vi "Get Protection Classes List.vi"(8 "error in (no error)":errorcluster) -> (0 "error out":errorcluster, 2 "Protection names":string[](array[string]), 3 "Class Lookup":variant)   [LabVIEW 2024, in "Instrument Addon Scripting API.lvlib"]
uses:
  Instrument Addon Scripting API.lvlib
  <vilib>/Utility/LVLibp/NI_PackedLibraryUtility.lvlib
  NationalInstruments.VeriStand
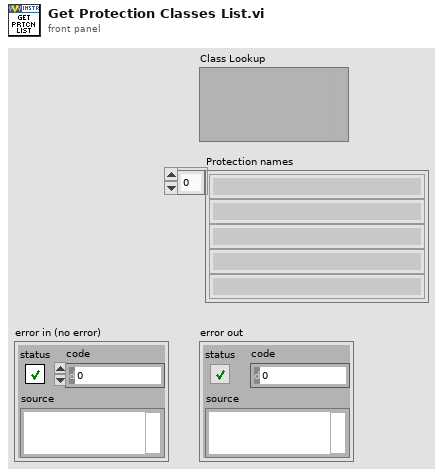
[diagram p1: front panel]
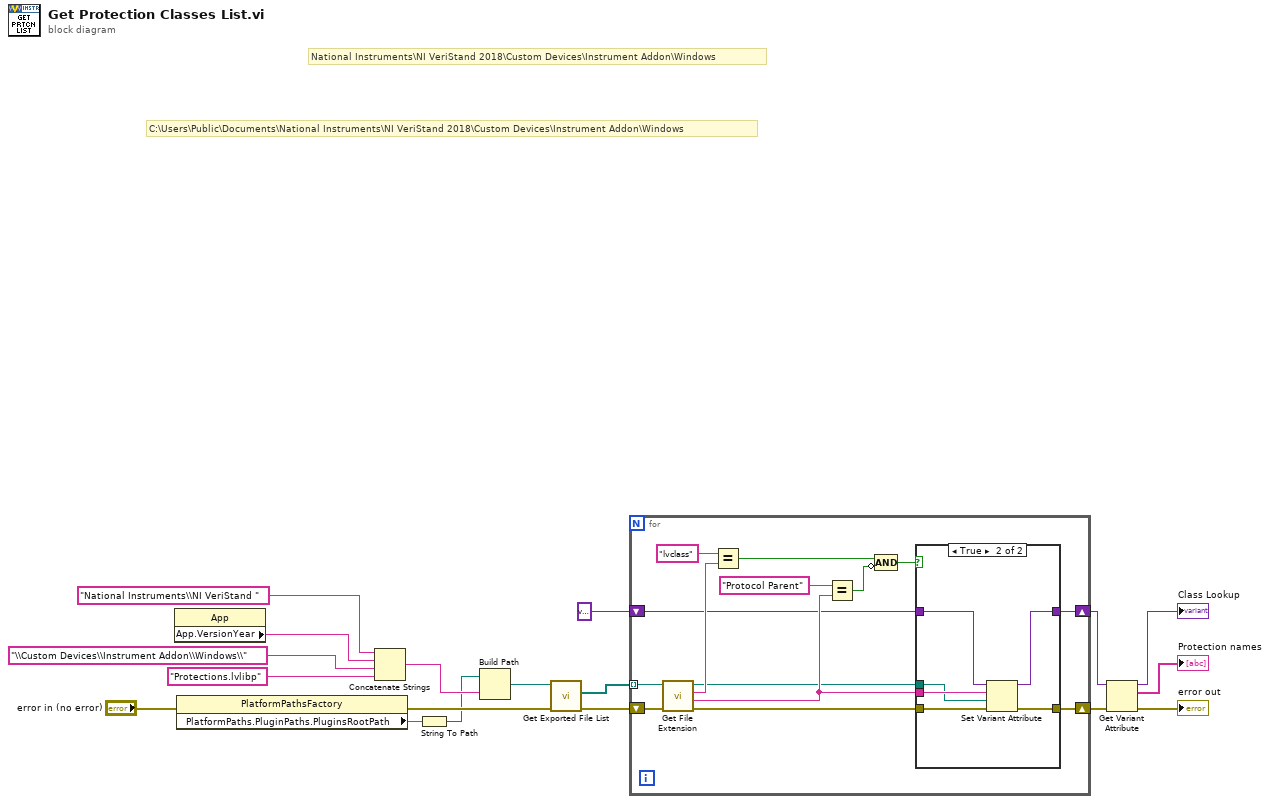
[diagram p0: block diagram]
diagram:
  # "National Instruments\\NI VeriStand 2018\\Custom Devices\\Instrument Addon\\Windows"
  # "C:\\Users\\Public\\Documents\\National Instruments\\NI VeriStand 2018\\Custom Devices\\Instrument Addon\\Windows"
  n1 = property class="App"() -> ("App.VersionYear"=w16:string)  [unwired: 2 in, 2 out]
  n2 = property class="PlatformPathsFactory"(error in="error in (no error)") -> (error out=w4:errorcluster, "PlatformPaths.PluginPaths.PluginsRootPath"=w2:string)  [unwired: 1 in, 1 out]
  n3 = Concatenate Strings("National Instruments\\NI VeriStand " ("string"), w16, "\\Custom Devices\\Instrument Addon\\Windows\\" ("string"), "Protections.lvlibp" ("name or relative path")) -> (w18:string)
  n4 = String To Path(string=w2) -> (path=w1:path)
  n5 = Build Path(base path=w1, name or relative path=w18) -> (appended path=w11:path)
  n6 = call <vilib>:"Get Exported File List.vi"("error in (no error)"=w4, "packed library path"=w11) -> ("error out"=w13:errorcluster, "paths"=w12:path[])  [unwired: 7 in, 1 out]
  n7 = for {
    tunnel: w12 -> [w27] mode=indexing
    shift-right: [w21] -> w8
    shift-left: w13 -> [w28]
    shift-right: [w20] -> w6
    shift-left: variant ("variant") -> [w23]
    n8 = call <vilib>:"Get File Extension.vi"("error in (no error)"=w28, "file"=w27) -> ("error out"=w22:errorcluster, "filename without extension"=w25:string, "lowercase file extension"=w29:string, "dup file"=w24:path)  [unwired: 5 in, 1 out]
    n9 = Equal?(x="lvclass" ("string"), y=w29) -> (x = y?=w31:bool)
    n10 = Equal?(x="Protocol Parent", y=w25) -> (x = y?=w26:bool)
    n11 = Compound Arithmetic op=AND(w31, invert w26) -> (w19:bool)
    n12 = case shown="True" w19 {
      tunnel: w25 -> [_ w40]
      tunnel: w24 -> [_ w39]
      tunnel: w23 -> [w33 w38]
      tunnel: w22 -> [w34 w37]
      tunnel: [w34 w36] -> w21
      tunnel: [w33 w35] -> w20
      frame False {
      }
      frame True {
        n13 = Set Variant Attribute(Variant=w38, name=w40, value=w39, error in=w37) -> (Variant out=w35:variant, error out=w36:errorcluster)  [unwired: 1 out]
      }
    }
  }
  n14 = Get Variant Attribute(Variant=w6, error in=w8) -> (duplicate Variant=→"Class Lookup":variant, names=→"Protection names":string[], error out=→"error out":errorcluster)  [unwired: 2 in, 1 out]
